vi "Angle Rotation (scalar).vi"(7 "angle units":T1 items=["radian in, radian out", "radian in, degree out", "degree in, degree out", "degree in, radian out"], 9 "rotated angle range":T2=1 items=["none", "-180 to 180 (-pi to pi)", "0 to 360 (0 to 2pi)"], 10 "counterclockwise rotation":dbl, 11 "angle":dbl) -> (0 "error":i32, 3 "rotated angle":dbl)   [LabVIEW 2020, in "NI_AAL_Angle.lvlib"]
doc: "Rotates the input angle counterclockwise.\n\nWire data to the angle input to determine the polymorphic instance to use or manually select the instance."
uses:
  <vilib>/Analysis/NI_AAL_Angle.lvlib
  <vilib>/Analysis/coordinate.llb/Angle Range (Degree).ctl
  <vilib>/Analysis/coordinate.llb/Angle Units.ctl
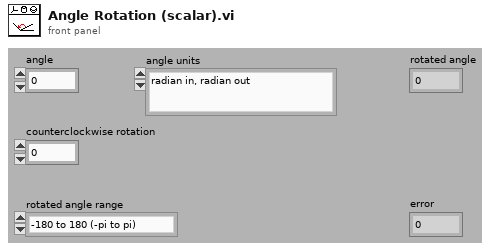
[diagram p1: front panel]
types:
  T1 = typedef "NI_AAL_Angle.lvlib/Angle Units.ctl" = i32
  T2 = typedef "NI_AAL_Angle.lvlib/Angle Range (Degree).ctl" = u16
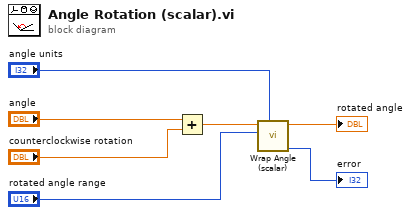
[diagram p0: block diagram]
diagram:
  n1 = Add(x="angle", y="counterclockwise rotation") -> (x+y=w5:dbl)
  n2 = call <vilib>:"Wrap Angle (scalar).vi"("angle units"="angle units", "angle range"="rotated angle range", "angle in"=w5) -> ("error"=→"error":i32, "angle out"=→"rotated angle":dbl)  [unwired: 7 in]
